vi "Show Description.vi"(8 "error in":errorcluster, 10 "Description":string, 11 "Peer Review in":refnum<class "Peer Review.lvclass">) -> (0 "error out":errorcluster, 3 "Peer Review out":refnum<class "Peer Review.lvclass">)   [LabVIEW 2020, in "Peer Review.lvclass"]
uses:
  Peer Review.lvclass
  Peer Review.lvclass/Peer Review.ctl
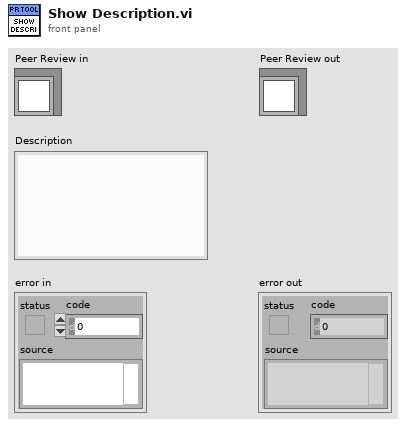
[diagram p1: front panel]
types:
  T1 = enum32{"Commit History", "File List", "Git Log", "Description", "Image"}
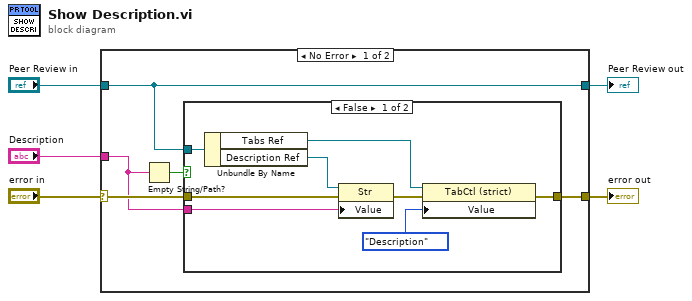
[diagram p0: block diagram]
diagram:
  n1 = case shown="No Error" "error in" {
    selector: "error in" -> [w9 w21]
    tunnel: [w7 w21] -> w4
    tunnel: [w10 w20] -> w2
    tunnel: "Peer Review in" -> [w10 w20]
    tunnel: "Description" -> [w8 _]
    frame No Error {
      n2 = Empty String/Path?(string/path=w8) -> (empty?=w6:bool)
      n3 = case shown="False" w6 {
        tunnel: w10 -> [w18 _]
        tunnel: w9 -> [w17 w19]
        tunnel: w8 -> [w15 _]
        tunnel: [w12 w19] -> w7
        frame False {
          n4 = Unbundle By Name(w18) -> ("Tabs Ref"=w13:refnum<vi>, "Description Ref"=w16:refnum<vi>)
          n5 = property class="Str"(reference=w16, error in=w17, "Value"=w15) -> (error out=w14:errorcluster)  [unwired: 1 out]
          n6 = property class="TabCtl (strict)"(reference=w13, error in=w14, "Value"=T1."Description") -> (error out=w12:errorcluster)  [unwired: 1 out]
        }
        frame True {
        }
      }
    }
    frame Error {
    }
  }
  "error out" <- w4
  "Peer Review out" <- w2
